vi "Create File.vi"() -> ()   [LabVIEW 2018]
uses:
  a872959d-f2d0-4aeb-a121-93ae34c04bb1.vi
  <vilib>/Utility/file.llb/Write Delimited Spreadsheet (string).vi
panel:
  out "shuffled array":string[](array[string])
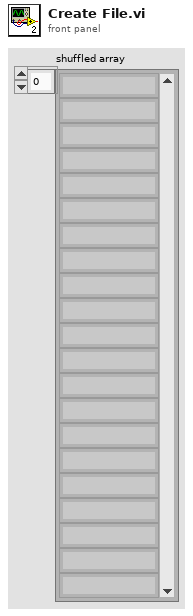
[diagram p1: front panel]
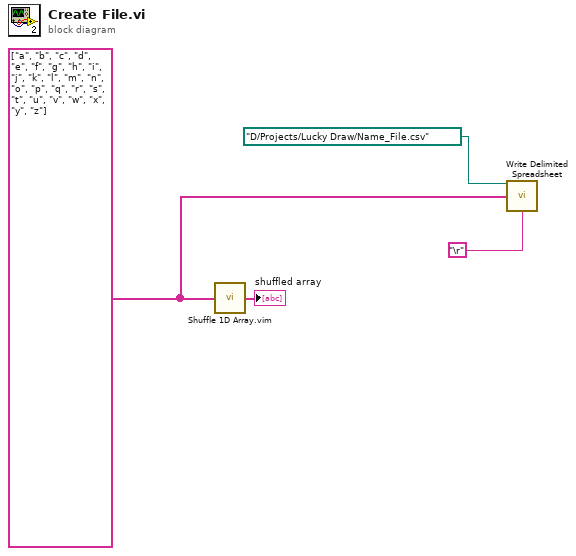
[diagram p0: block diagram]
diagram:
  w3 = string[] ["a", "b", "c", "d", "e", "f", "g", "h", "i", "j", "k", "l", "m", "n", "o", "p", "q", "r", "s", "t", "u", "v", "w", "x", "y", "z"]
  n1 = call "Shuffle 1D Array.vim"("array"=w3) -> ("shuffled array"=→"shuffled array":string[])  [unwired: 4 in]
  n2 = call-poly <vilib>:"Write Delimited Spreadsheet.vi"("file path (dialog if empty)"=path "D:/Projects/Lucky Draw/Name_File.csv", "1D data"=w3, "delimiter (\\t)"="\r") -> ()  [unwired: 11 in, 2 out]
